vi "Set PID Control.vi"(10 "PID Control":bool, 11 "arm in":refnum<class "arm.lvclass">) -> (3 "arm out":refnum<class "arm.lvclass">)   [LabVIEW 2015, in "arm.lvclass"]
uses:
  arm.lvclass
  arm.lvclass/arm.ctl
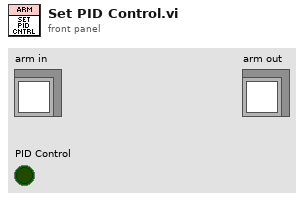
[diagram p1: front panel]
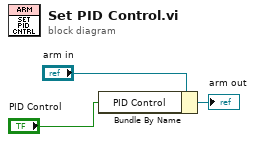
[diagram p0: block diagram]
diagram:
  n1 = Bundle By Name(cluster="arm in", "PID Control"="PID Control") -> (→"arm out":refnum<class "arm.lvclass">)
